vi "Tanques 1.vi"() -> ()   [LabVIEW 2020]
panel:
  in  "Slide 2":i32(slide) scale=0.0..10.0
  in  "Slide":i32(slide) scale=0.0..10.0
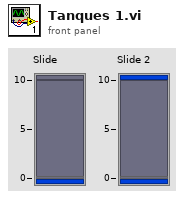
[diagram p1: front panel]
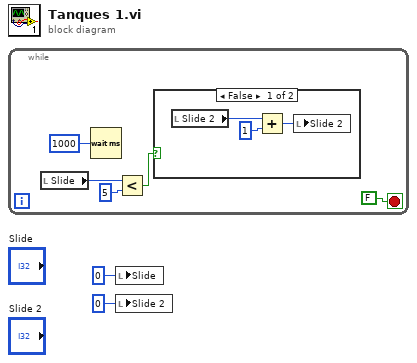
[diagram p0: block diagram]
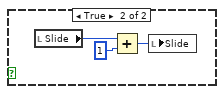
[diagram p2: hidden frame]
diagram:
  n1 = while {
    stop <- FALSE stop-if-true
    n2 = local read "Slide"() -> (w6:i32)
    n3 = Wait (ms)(milliseconds to wait=u32 1000) -> ()  [unwired: 1 out]
    n4 = Less?(x=w6, y=5) -> (x < y?=w5:bool)
    n5 = case shown="False" w5 {
      frame False {
        n6 = local read "Slide 2"() -> (w9:i32)
        n7 = Add(x=w9, y=1) -> (x+y=w10:i32)
        n8 = local write "Slide 2"(w10) -> ()
      }
      frame True {
        n9 = local read "Slide"() -> (w12:i32)
        n10 = Add(x=w12, y=1) -> (x+y=w13:i32)
        n11 = local write "Slide"(w13) -> ()
      }
    }
  }
  n12 = local write "Slide"(0 ("Slide")) -> ()
  n13 = local write "Slide 2"(0 ("Slide 2")) -> ()
